vi "RFFE Extended Register Read Example.vi"() -> ()   [LabVIEW 2018]
uses:
  Slave Address.ctl
  Register Address.ctl
  Register Data.ctl
  MIPI RFFE API.lvlib
panel:
  out "Register Data":T1[](array[typedef]) format="%02x"
  in  "Byte Count":i32=1
  in  "Register Address":T2 format="%02x"
  in  "Slave Address":T3=12 format="%02x"
  in  "Bus Number":i32
  in  "Resource Name":refnum<k15>
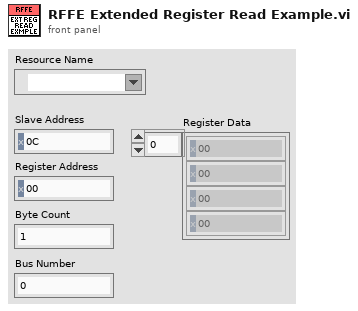
[diagram p1: front panel]
types:
  T1 = typedef "MIPI RFFE API.lvlib/Register Data.ctl" = u8
  T2 = typedef "MIPI RFFE API.lvlib/Register Address.ctl" = u16
  T3 = typedef "MIPI RFFE API.lvlib/Slave Address.ctl" = u8
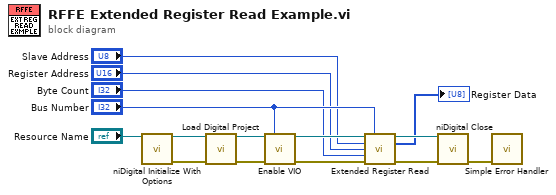
[diagram p0: block diagram]
diagram:
  n1 = call <instrlib>:"niDigital Initialize With Options.vi"("resource name"="Resource Name") -> ("instrument handle"=w7:refnum<k15>, "error out"=w6:errorcluster)  [unwired: 13 in]
  n2 = call "Load Digital Project.vi"("instrument handle"=w7, "error in"=w6) -> ("instrument handle out"=w15:refnum<k15>, "error out"=w14:errorcluster)  [unwired: 12 in]
  n3 = call "Enable VIO.vi"("instrument handle"=w15, "Bus Number"="Bus Number", "error in"=w14) -> ("instrument handle out"=w11:refnum<k15>, "error out"=w9:errorcluster)  [unwired: 11 in]
  n4 = call "Extended Register Read.vi"("instrument handle in"=w11, "Bus Number"="Bus Number", "Slave Address"="Slave Address", "Register Address"="Register Address", "Byte Count"="Byte Count", "error in (no error)"=w9) -> ("instrument handle out"=w10:refnum<k15>, "Register Data"=→"Register Data":T1[], "error out"=w8:errorcluster)  [unwired: 7 in]
  n5 = call <instrlib>:"niDigital Close.vi"("instrument handle"=w10, "error in"=w8) -> ("error out"=w12:errorcluster)  [unwired: 13 in]
  n6 = call <vilib>:"Simple Error Handler.vi"("error in (no error)"=w12) -> ()  [unwired: 4 in, 5 out]
